vi "Init.vi"(8 "error in (no error)":errorcluster, 9 "Replication Rounds":u32, 10 "Size":i32) -> (0 "error out":errorcluster, 3 "Map out":refnum<class "Map.lvclass">)   [LabVIEW 2020, in "SquareBattle.lvlib" / "Map.lvclass"]
uses:
  Map.lvclass
  Square/Square.lvclass
  Run Result.ctl
  Action.ctl
  Direction.ctl
  Map.lvclass/Map.ctl
  SquareBattle.lvlib
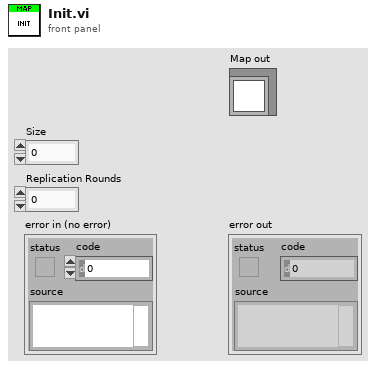
[diagram p1: front panel]
types:
  T1 = typedef "SquareBattle.lvlib/Run Result.ctl" = cluster{"Action":T2, "Direction":T3, "Replication":refnum<class "Square.lvclass">}
  T2 = typedef "SquareBattle.lvlib/Action.ctl" = enum16{"Wait", "Move", "Attack", "Replicate"}
  T3 = typedef "SquareBattle.lvlib/Direction.ctl" = enum16{"NW", "N", "NE", "E", "SE", "S", "SW", "W"}
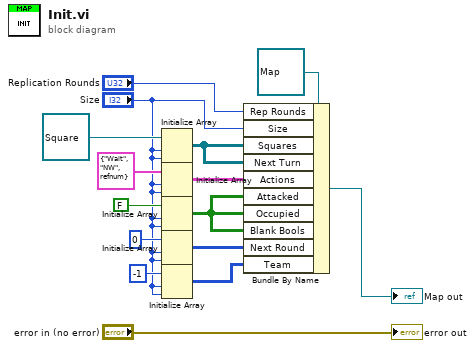
[diagram p0: block diagram]
diagram:
  n1 = Initialize Array(refnum<class "Square.lvclass"> refnum ("SquareBattle:Square"), "Size", "Size") -> (w2:refnum<class "Square.lvclass">[][])
  n2 = Initialize Array(T1 {"Action"=enum."Wait", "Direction"=enum."NW", "Replication"=refnum} ("Run Result"), "Size", "Size") -> (w11:T1[][])
  n3 = Initialize Array(FALSE, "Size", "Size") -> (w1:bool[][])
  n4 = Initialize Array(u32 0, "Size", "Size") -> (w7:u32[][])
  n5 = Initialize Array(-1, "Size", "Size") -> (w5:i32[][])
  n6 = Bundle By Name(cluster=refnum<class "Map.lvclass"> refnum ("Map in"), "Rep Rounds"="Replication Rounds", "Size"="Size", "Squares"=w2, "Next Turn"=w2, "Actions"=w11, "Attacked"=w1, "Occupied"=w1, "Blank Bools"=w1, "Next Round"=w7, "Team"=w5) -> (→"Map out":refnum<class "Map.lvclass">)
  "error out" <- "error in (no error)"
